vi "PanelUpdates_Enable.vi"(8 "error in (no error)":errorcluster, 11 "Parent VI Reference":refnum<vi>) -> (0 "error out":errorcluster)   [LabVIEW 2014, in "hse-ui.lvlib"]
doc: "____\nHAMPEL SOFTWARE ENGINEERING v0.7.0 (2018-07-16 18:12)"
uses:
  hse-ui.lvlib
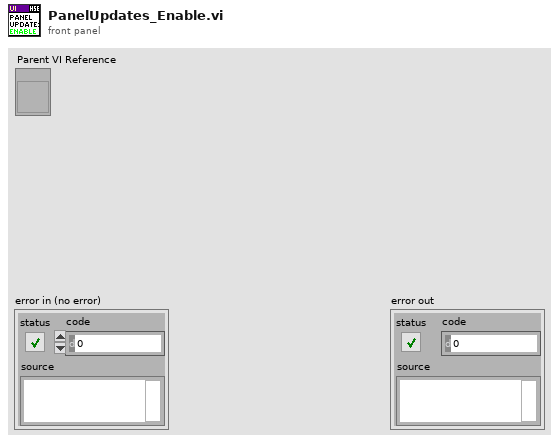
[diagram p1: front panel]
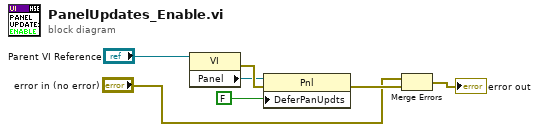
[diagram p0: block diagram]
diagram:
  n1 = property class="VI"(reference="Parent VI Reference") -> (error out=w5:errorcluster, "Panel"=w4:refnum<vi>)  [unwired: 1 in, 1 out]
  n2 = property class="Pnl"(reference=w4, error in=w5, "DeferPanUpdts"=FALSE ("Defer Panel Updates")) -> (error out=w3:errorcluster)  [unwired: 1 out]
  n3 = Merge Errors("error in (no error)", w3) -> (→"error out":errorcluster)
